vi "Check status -- subVI.vi"(8 "error in (no error)":errorcluster, 11 "Input string":string="1TS00000A") -> (0 "error out":errorcluster, 3 "Controller state":T1)   [LabVIEW 2020, in "FCR100.lvlib"]
uses:
  FCR100.lvlib
  Controller state -- enum.ctl
  <vilib>/Utility/error.llb/Error Cluster From Error Code.vi
  <vilib>/ErrorRing/Error Ring.xnode
panel:
  out "Error arr":string[](array[string])
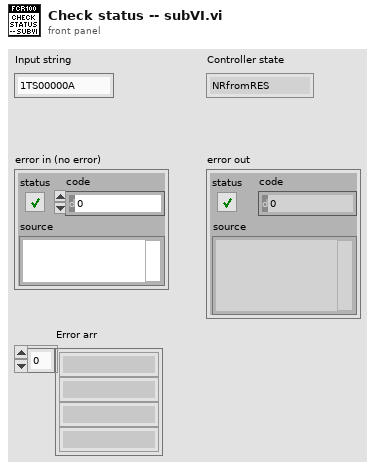
[diagram p1: front panel]
types:
  T1 = typedef "Controller state -- enum.ctl" = enum16{"NRfromRES", "NRfromHOM", "NRfromCONF", "NRfromDIS", "NRfromRDY", "NRfromMOV", "NR-NPM", "CONFIG", "HOMING", "MOVING", "RDYfromHOM", "RDYfromMOV", "RDYfromDIS", "DISfromRDY", "DISfromMOV"}
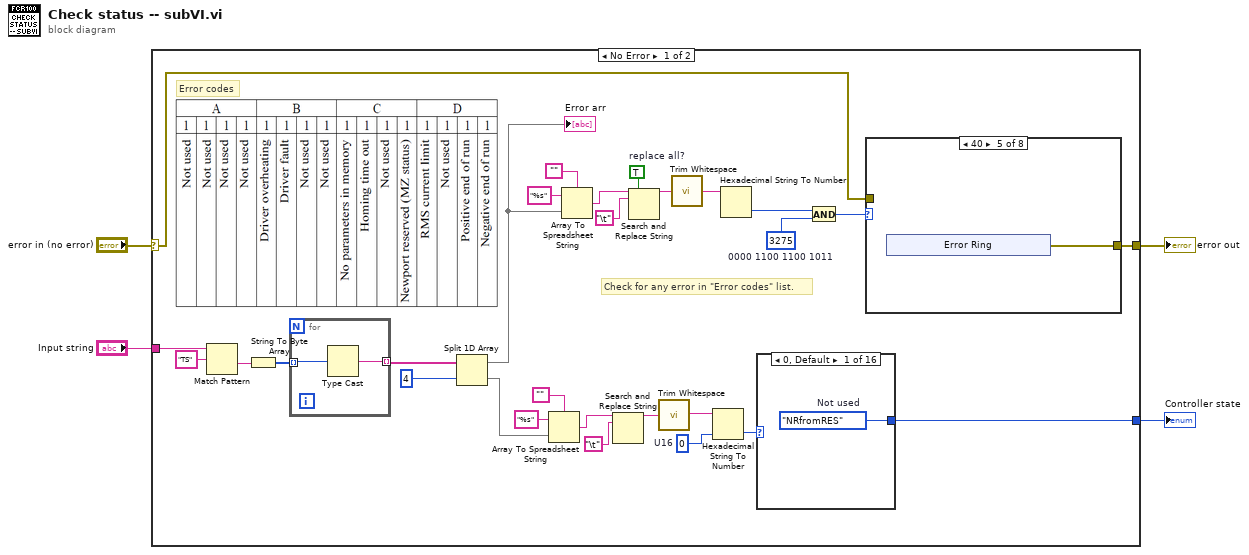
[diagram p0: block diagram]
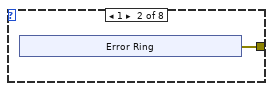
[diagram p3: hidden frame]
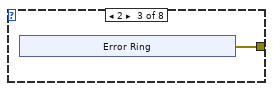
[diagram p4: hidden frame]
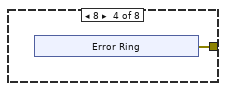
[diagram p5: hidden frame]
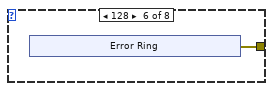
[diagram p6: hidden frame]
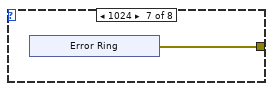
[diagram p7: hidden frame]
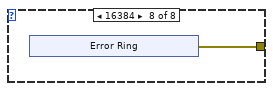
[diagram p8: hidden frame]
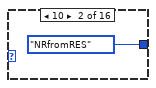
[diagram p9: hidden frame]
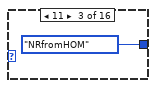
[diagram p10: hidden frame]
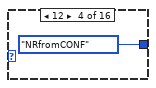
[diagram p11: hidden frame]
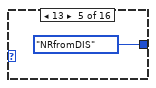
[diagram p12: hidden frame]
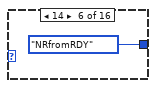
[diagram p13: hidden frame]
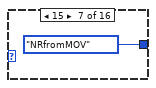
[diagram p14: hidden frame]
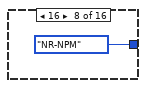
[diagram p15: hidden frame]
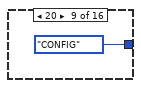
[diagram p16: hidden frame]
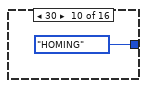
[diagram p17: hidden frame]
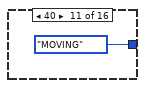
[diagram p18: hidden frame]
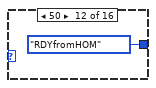
[diagram p19: hidden frame]
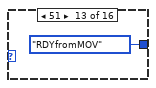
[diagram p20: hidden frame]
diagram:
  n1 = case shown="No Error" "error in (no error)" {
    selector: "error in (no error)" -> [w6 w96]
    tunnel: "Input string" -> [w32 _]
    tunnel: [w7 Controller_state_--_enum."NR-NPM" ("Controller states")] -> w2
    tunnel: [w5 w96] -> w1
    frame No Error {
      w9 = TRUE  # replace all?
      w17 = u32 3275  # 0000 1100 1100 1011
      w20 = u16 0  # U16
      # "Error codes"
      # "Check for any error in \"Error codes\" list."
      n2 = Match Pattern(string=w32, regular expression="TS") -> (after substring=w31:string)  [unwired: 1 in, 3 out]
      n3 = String To Byte Array(string=w31) -> (unsigned byte array=w30:u8[])
      n4 = for {
        tunnel: w30 -> [w94] mode=indexing
        tunnel: [w93] -> w29 mode=indexing
        n5 = Type Cast(x=w94) -> (*(type *) &x=w93:string)  [unwired: 1 in]
      }
      n6 = Split 1D Array(array=w29, index=4) -> (first subarray=w12:string[], second subarray=w27:string[])
      "Error arr" <- w12
      n7 = Array To Spreadsheet String(delimiter (Tab)="", array=w27, 3:"%s" ("format string")) -> (spreadsheet string=w24:string)
      n8 = Array To Spreadsheet String(delimiter (Tab)="", array=w12, 3:"%s" ("format string")) -> (spreadsheet string=w15:string)
      n9 = Search and Replace String(input string=w24, search string="\t") -> (result string=w22:string)  [unwired: 6 in, 3 out]
      n10 = Search and Replace String(replace all?=w9, input string=w15, search string="\t") -> (result string=w16:string)  [unwired: 5 in, 3 out]
      n11 = call <vilib>:"Trim Whitespace.vi"("string"=w22) -> ("trimmed string"=w21:string)  [unwired: 1 in]
      n12 = call <vilib>:"Trim Whitespace.vi"("string"=w16) -> ("trimmed string"=w11:string)  [unwired: 1 in]
      n13 = Hexadecimal String To Number(string=w21, default (0uL)=w20) -> (number=w19:u16)  [unwired: 1 in, 1 out]
      n14 = Hexadecimal String To Number(string=w11) -> (number=w18:u32)  [unwired: 2 in, 1 out]
      n15 = case shown="0, Default" w19 {
        tunnel: [w77 Controller_state_--_enum."NRfromRES" ("Controller states") Controller_state_--_enum."NRfromHOM" ("Controller states") Controller_state_--_enum."NRfromCONF" ("Controller states") Controller_state_--_enum."NRfromDIS" ("Controller states") Controller_state_--_enum."NRfromRDY" ("Controller states") Controller_state_--_enum."NRfromMOV" ("Controller states") Controller_state_--_enum."NR-NPM" ("Controller states") Controller_state_--_enum."CONFIG" ("Controller states") Controller_state_--_enum."HOMING" ("Controller states") Controller_state_--_enum."MOVING" ("Controller states") Controller_state_--_enum."RDYfromHOM" ("Controller states") Controller_state_--_enum."RDYfromMOV" ("Controller states") Controller_state_--_enum."RDYfromDIS" ("Controller states") Controller_state_--_enum."DISfromRDY" ("Controller states") Controller_state_--_enum."DISfromMOV" ("Controller states")] -> w7
        frame 0, Default {
          w77 = Controller_state_--_enum."NRfromRES"  # Not used
        }
        frame 10 {
        }
        frame 11 {
        }
        frame 12 {
        }
        frame 13 {
        }
        frame 14 {
        }
        frame 15 {
        }
        frame 16 {
        }
        frame 20 {
        }
        frame 30 {
        }
        frame 40 {
        }
        frame 50 {
        }
        frame 51 {
        }
        frame 52 {
        }
        frame 60 {
        }
        frame 61 {
        }
      }
      n16 = And(x=w18, y=w17) -> (x .and. y?=w8:u32)
      n17 = case shown="40" w8 {
        tunnel: w6 -> [w34 _ _ _ _ _ _ _]
        tunnel: [w34 w35 w41 w47 w53 w59 w65 w71] -> w5
        frame 0, Default {
        }
        frame 1 {
          n18 = xnode "Error Ring"() -> ("error out"=w35:errorcluster)
        }
        frame 2 {
          n19 = xnode "Error Ring"() -> ("error out"=w41:errorcluster)
        }
        frame 8 {
          n20 = xnode "Error Ring"() -> ("error out"=w47:errorcluster)
        }
        frame 64 {
          n21 = xnode "Error Ring"() -> ("error out"=w53:errorcluster)
        }
        frame 128 {
          n22 = xnode "Error Ring"() -> ("error out"=w59:errorcluster)
        }
        frame 1024 {
          n23 = xnode "Error Ring"() -> ("error out"=w65:errorcluster)
        }
        frame 16384 {
          n24 = xnode "Error Ring"() -> ("error out"=w71:errorcluster)
        }
      }
    }
    frame Error {
    }
  }
  "Controller state" <- w2
  "error out" <- w1
